vi "SUB_RunTime_FilePath.vi"() -> (1 "stripped path":path)   [LabVIEW 2011]
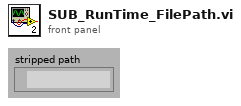
[diagram p1: front panel]
types:
  T1 = enum32{"invalid app kind", "Development System", "Run Time System", "Student Edition", "Embedded LabVIEW", "Evaluation", "Custom"}
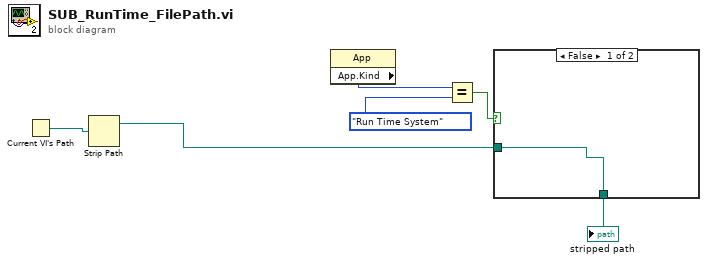
[diagram p0: block diagram]
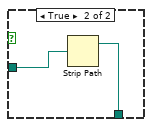
[diagram p2: hidden frame]
diagram:
  n1 = Current VI's Path() -> (path=w6:path)
  n2 = Strip Path(path=w6) -> (stripped path=w2:path)  [unwired: 1 out]
  n3 = property class="App"() -> ("App.Kind"=w5:T1)  [unwired: 2 in, 2 out]
  n4 = Equal?(x=w5, y=T1."Run Time System" ("Application:Kind")) -> (x = y?=w3:bool)
  n5 = case shown="False" w3 {
    tunnel: w2 -> [w7 w9]
    tunnel: [w7 w8] -> w1
    frame False {
    }
    frame True {
      n6 = Strip Path(path=w9) -> (stripped path=w8:path)  [unwired: 1 out]
    }
  }
  "stripped path" <- w1
